vi "Average PSI FGV.vi"(10 "Current Pressure.":i32, 11 "Average On?":bool) -> (2 "Average Pressure":i32)   [LabVIEW 2013]
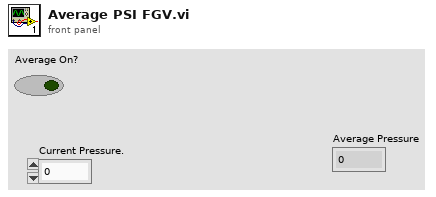
[diagram p1: front panel]
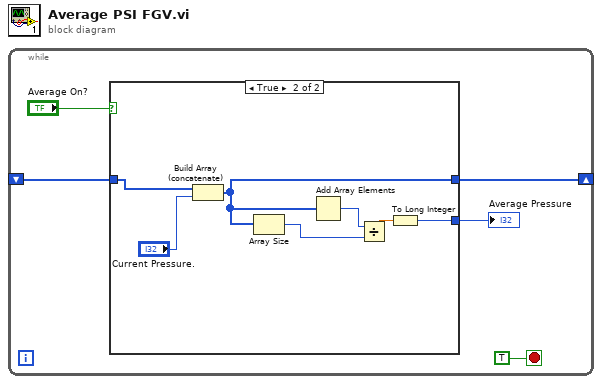
[diagram p0: block diagram]
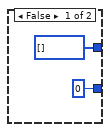
[diagram p2: hidden frame]
diagram:
  n1 = while {
    shift-right: [w3] -> _
    shift-left: _ -> [w2]
    stop <- TRUE stop-if-true
    n2 = case shown="True" "Average On?" {
      tunnel: [i32[] [] w12] -> w3
      tunnel: w2 -> [_ w13]
      tunnel: [0 w8] -> w1
      frame False {
      }
      frame True {
        n3 = Build Array (concatenate)(w13, "Current Pressure.") -> (w12:i32[])
        n4 = Array Size(array=w12) -> (size(s)=w10:i32)
        n5 = Add Array Elements(numeric array=w12) -> (sum=w11:i32)
        n6 = Divide(x=w11, y=w10) -> (x/y=w9:dbl)
        n7 = To Long Integer(number=w9) -> (32bit integer=w8:i32)
      }
    }
    "Average Pressure" <- w1
  }
